vi "_Destroy.vi"(8 "error in (no error)":errorcluster, 11 "Std Dev in":refnum<class "Std Dev.lvclass">) -> (0 "error out":errorcluster)   [LabVIEW 2009, in "Std Dev.lvclass"]
uses:
  Std Dev.lvclass
  Readable/Readable.lvclass
  Std Dev.lvclass/Std Dev.ctl
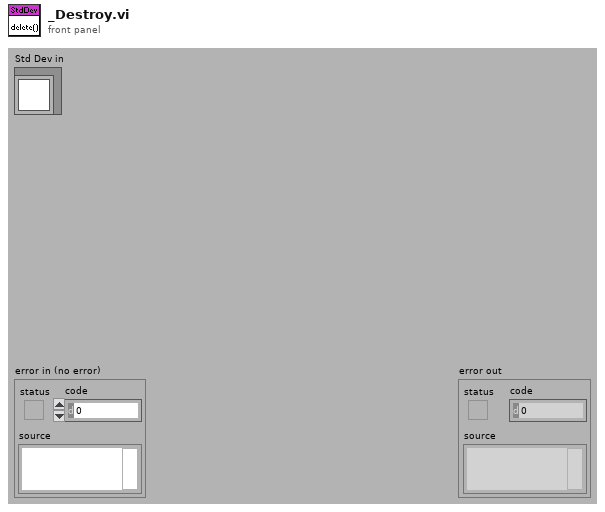
[diagram p1: front panel]
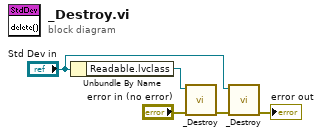
[diagram p0: block diagram]
diagram:
  n1 = Unbundle By Name("Std Dev in") -> ("Readable.lvclass"=w3:refnum<class "Readable.lvclass">)
  n2 = call-dynamic "_Destroy.vi"("error in (no error)"="error in (no error)", "Instrument in"=w3) -> ("error out"=w1:errorcluster)  [unwired: 9 out]
  n3 = call-parent "_Destroy.vi"("error in (no error)"=w1, "Instrument in"="Std Dev in") -> ("error out"=→"error out":errorcluster)  [unwired: 9 out]
